vi "Merge.vi"(9 "element in":T1, 10 "lastWrtIdx in":i32, 11 "array in":cluster{"elt":T1}[](array[cluster])) -> (2 "lastWrtIdx out":i32, 3 "array out":cluster{"elt":T1}[](array[cluster]), 5 "merged?":bool)   [LabVIEW 2019, in "MessengerM.lvlib" / "SubChannelCPU.lvclass"]
uses:
  SubChannelCPU.lvclass
  <vilib>/ChannelSupport/Channel Message/Channel Message.lvclass
  Element.ctl
  MessengerM.lvlib
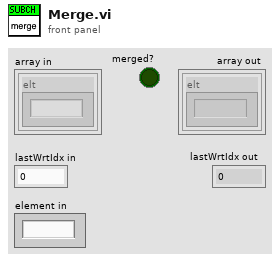
[diagram p1: front panel]
types:
  T1 = typedef "MessengerM.lvlib/Element.ctl" = string
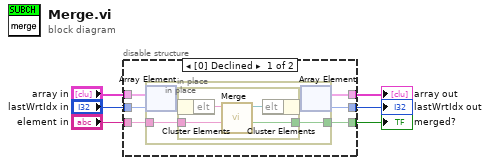
[diagram p0: block diagram]
diagram:
  n1 = disable-structure shown="[0] Declined" {
    disable-tunnel: "array in" -> [w12 w22]
    disable-tunnel: [w11 w22] -> w2
    disable-tunnel: [w10 _] -> w3
    disable-tunnel: "lastWrtIdx in" -> [w9 w21]
    disable-tunnel: [w8 w21] -> w5
    disable-tunnel: "element in" -> [w7 _]
    frame Disabled {
      n2 = in-place {
        in-place-border: w7 -> [w16]
        in-place-border: [w15] -> w10
        n3 = in-place-array #1(w12, w9) -> (w14:cluster{"elt":T1})
        n4 = in-place {
          in-place-border: w16 -> [w20]
          in-place-border: [w19] -> w15
          n5 = in-place-cluster #2(w14) -> ("elt"=w17:T1)
          n6 = call-dynamic "Merge.vi"("new message"=w20, "already enqueued message"=w17) -> ("merged?"=w19:bool, "merged message"=w18:refnum<class "Channel Message.lvclass">)  [unwired: 8 in]
          n7 = in-place-cluster #2("elt"=w18) -> (w13:cluster{"elt":T1})
        }
        n8 = in-place-array #1(w13) -> (w11:cluster{"elt":T1}[], w8:i32)
      }
    }
    frame Enabled {
    }
  }
  "lastWrtIdx out" <- w5
  "merged?" <- w3
  "array out" <- w2
